vi "SetStagePosition.vi"(0 "StageController in":refnum<class "StageController.lvclass">, 5 "Label":string, 7 "AbsPosition?":bool=TRUE, 9 "Value":dbl format="%#_13g", 11 "error in (no error)":errorcluster) -> (4 "StageController out":refnum<class "StageController.lvclass">, 15 "error out":errorcluster)   [LabVIEW 2020, in "StageController.lvclass"]
uses:
  StageController.lvclass
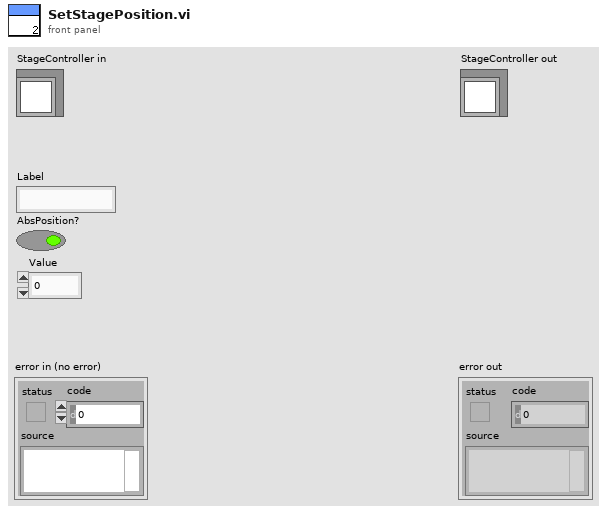
[diagram p1: front panel]
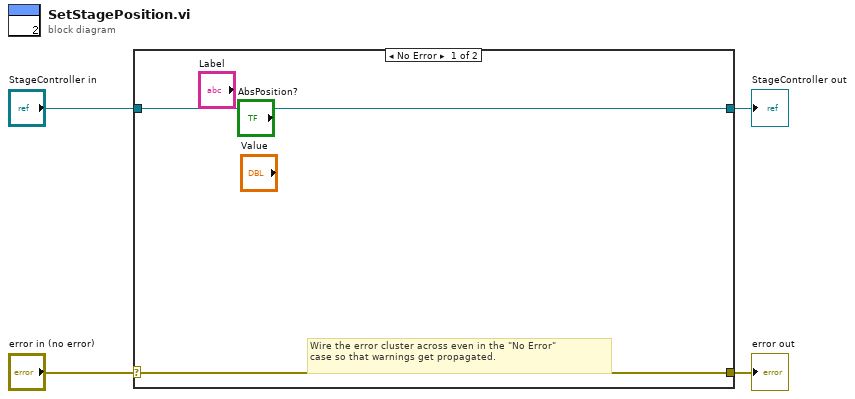
[diagram p0: block diagram]
diagram:
  n1 = case shown="No Error" "error in (no error)" {
    selector: "error in (no error)" -> [w5 w8]
    tunnel: [w5 w8] -> w3
    tunnel: [w6 w7] -> w1
    tunnel: "StageController in" -> [w6 w7]
    frame No Error {
      # "Wire the error cluster across even in the \"No Error\"\ncase so that warnings get propagated."
    }
    frame Error {
    }
  }
  "error out" <- w3
  "StageController out" <- w1
